vi "Add Entry.vi"(0 "Tree Map in":refnum<class "Tree Map.lvclass">, 1 "Symbol":string, 2 "BG Color (None)":u32(colorbox), 5 "Name":string, 7 "Name Prefix (none)":string, 9 "Columns":string[](array[string]), 11 "error in":errorcluster, 12 "Parent (None)":string[](array[string])) -> (4 "Tree Map out":refnum<class "Tree Map.lvclass">, 14 "Hierarchy":string[](array[string]), 15 "error out":errorcluster)   [LabVIEW 2026, in "Tree Map.lvlib" / "Tree Map.lvclass"]
uses:
  Tree Map.lvclass
  Tree Entry.ctl
  Tree Map.lvclass/Tree Map.ctl
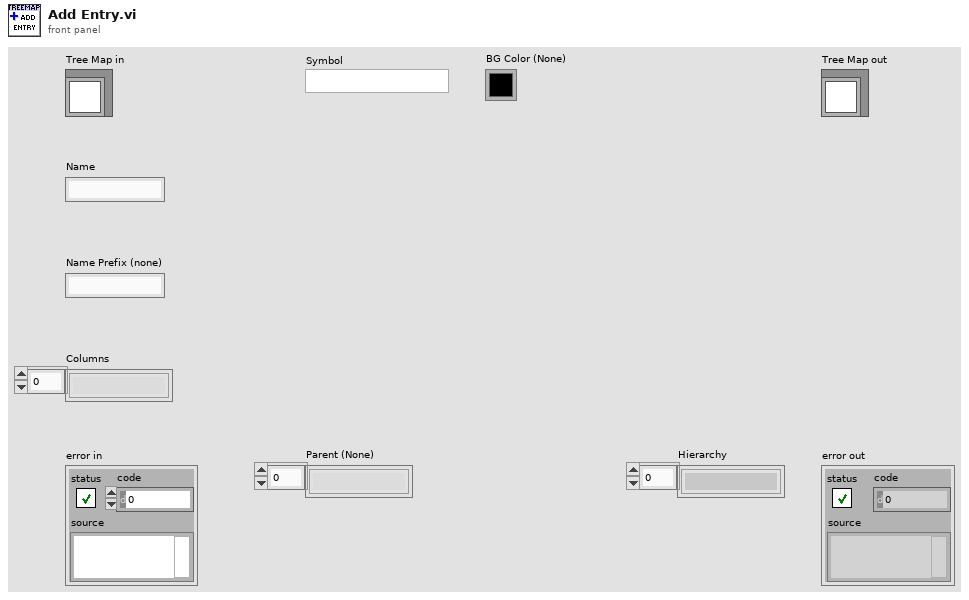
[diagram p1: front panel]
types:
  T1 = typedef "Tree Map.lvlib/Tree Map.lvclass/Tree Entry.ctl" = cluster{"Hierarchy":string[], "Name":string, "Columns":string[], "BG Color":u32, "Leaf":bool, "Symbol":string}
  T2 = typedef "imagedata.ctl" = cluster{"image type":i32, "image depth":i32, "image":u8[], "mask":u8[], "colors":u32[], "Rectangle":cluster{"left":i16, "top":i16, "right":i16, "bottom":i16}}
  T3 = map{string, cluster{"index":i32, "image data":T2}}
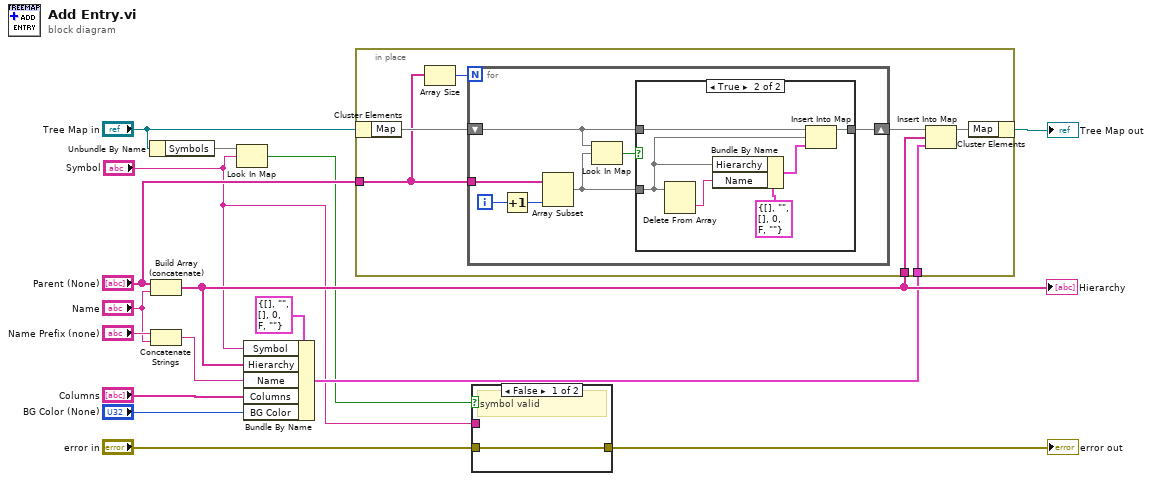
[diagram p0: block diagram]
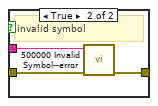
[diagram p2: hidden frame]
diagram:
  n1 = Unbundle By Name("Tree Map in") -> ("Symbols"=w6:T3)
  n2 = Build Array (concatenate)("Parent (None)", "Name") -> (w11:string[])
  "Hierarchy" <- w11
  n3 = Concatenate Strings("Name Prefix (none)", "Name") -> (w13:string)
  n4 = Look In Map(map=w6, key="Symbol") -> (key not found?=w2:bool)  [unwired: 1 in, 1 out]
  n5 = Bundle By Name(cluster=T1 {"Hierarchy"=[], "Name"="", "Columns"=[], "BG Color"=0, "Leaf"=FALSE, "Symbol"=""} ("Tree Entry"), "Symbol"="Symbol", "Hierarchy"=w11, "Name"=w13, "Columns"="Columns", "BG Color"="BG Color (None)") -> (w4:T1)
  n6 = in-place {
    in-place-border: w4 -> [w23]
    in-place-border: w11 -> [w22]
    in-place-border: "Parent (None)" -> [w18]
    n7 = in-place-cluster #1("Tree Map in") -> ("Map"=w20:map{string[], T1})
    n8 = Array Size(array=w18) -> (size(s)=w17:i32)
    n9 = for {
      N: w17 -> [_]
      shift-right: [w25] -> w19
      shift-left: w20 -> [w27]
      tunnel: w18 -> [w30]
      i -> [w29]
      n10 = Increment(x=w29) -> (x+1=w24:i32)
      n11 = Array Subset(array=w30, length=w24) -> (w26:string[])  [unwired: 1 in]
      n12 = Look In Map(map=w27, key=w26) -> (key not found?=w28:bool)  [unwired: 1 in, 1 out]
      n13 = case shown="True" w28 {
        tunnel: w27 -> [w31 w37]
        tunnel: w26 -> [_ w33]
        tunnel: [w31 w36] -> w25
        frame False {
        }
        frame True {
          n14 = Delete From Array(array=w33) -> (deleted portion=w32:string)  [unwired: 2 in, 1 out]
          n15 = Bundle By Name(cluster=T1 {"Hierarchy"=[], "Name"="", "Columns"=[], "BG Color"=0, "Leaf"=FALSE, "Symbol"=""} ("value"), "Hierarchy"=w33, "Name"=w32) -> (w34:T1)
          n16 = Insert Into Map(map in=w37, key=w33, value=w34) -> (map out=w36:map{string[], T1})  [unwired: 2 out]
        }
      }
    }
    n17 = Insert Into Map(map in=w19, key=w22, value=w23) -> (map out=w21:map{string[], T1})  [unwired: 2 out]
    n18 = in-place-cluster #1("Map"=w21) -> (→"Tree Map out":refnum<class "Tree Map.lvclass">)
  }
  n19 = case shown="False" w2 {
    tunnel: "error in" -> [w38 w41]
    tunnel: [w38 w40] -> w3
    tunnel: "Symbol" -> [_ w39]
    frame False {
      # "symbol valid"
    }
    frame True {
      # "invalid symbol"
      n20 = call "500000 Invalid Symbol--error.vi"("error in"=w41, "Argument"=w39) -> ("error out"=w40:errorcluster)  [unwired: 8 in, 1 out]
    }
  }
  "error out" <- w3
